vi "Fits_Create_Header.vi"(1 "Commentaire":string, 2 "Exptim":sgl, 3 "naxis3":i32=1, 4 "naxis2":i32, 5 "naxis1":i32, 6 "Type de données":T1) -> (0 "FITS header":string="SIMPLE  =                    T / Std FITS                                       BITPIX  =                    8 / NBER OF BITS PER PIXEL                         NAXIS   =                    2 / NBER OF AXIS                                   NAXIS1  =                    0 / FIRST VARYING AXIS                             NAXIS2  =                    0 / SECOND VARYING AXIS                            BZERO   =                    0 / DATA = BSCALE * DATA + BZERO                   BSCALE  =                    1 / DATA = BSCALE * DATA + BZERO                   DATE    =           11/03/2013 / LOCAL DATE dd/mm/yyyy                          TIME    =             11:26:53 / LOCAL TIME hh:mm:ss                            EXPTIM  =             0,000000 / INTEGRATION TIME  s                            NOM_PATI=               Durand / Nom du patient                                 COMMENT =                                                                                                                                                                                                                                       END                                                                                                                                                                                                                                                                                                                                                                                                                                                                                                                                                                                                                                                                                                                                                                                                                                                                                                                                                                                                                                                                                                                                                                                                                                                                                                                                                                                                                                                                                                                                                                                                                                                                                                                                                                                                                             ")   [LabVIEW 2020]
doc: "Creates the header string (multiple of 2880 characters) for a FITS image.\n\nThe dimensions of the data cube must be provided in input : they are naxis1, naxis2, naxis3. For a single image, set naxis3 to 1 (or any integer value less or equal to 1).\n\nThe data-types are:\n0 for U8 (unsigned 8bit)\n1 for I16 (signed integer 16bit)\n2 for I32 (signed integer 32bit)\n3 for SGL (float 32bit)\n4 for DBL(float 64bit)\n5 for complex (2xfloat 64bit)"
uses:
  DataTyp_Header.ctl
panel:
  in  "NomChamp":string="NOM_PATI"
  in  "Commentaire":string="Nom du patient"
  in  "VeleuChamp 1":string="Durand"
  out "FITS header 2":string
  in  "length (rest)":i32
  out "nb char header":i32=2880
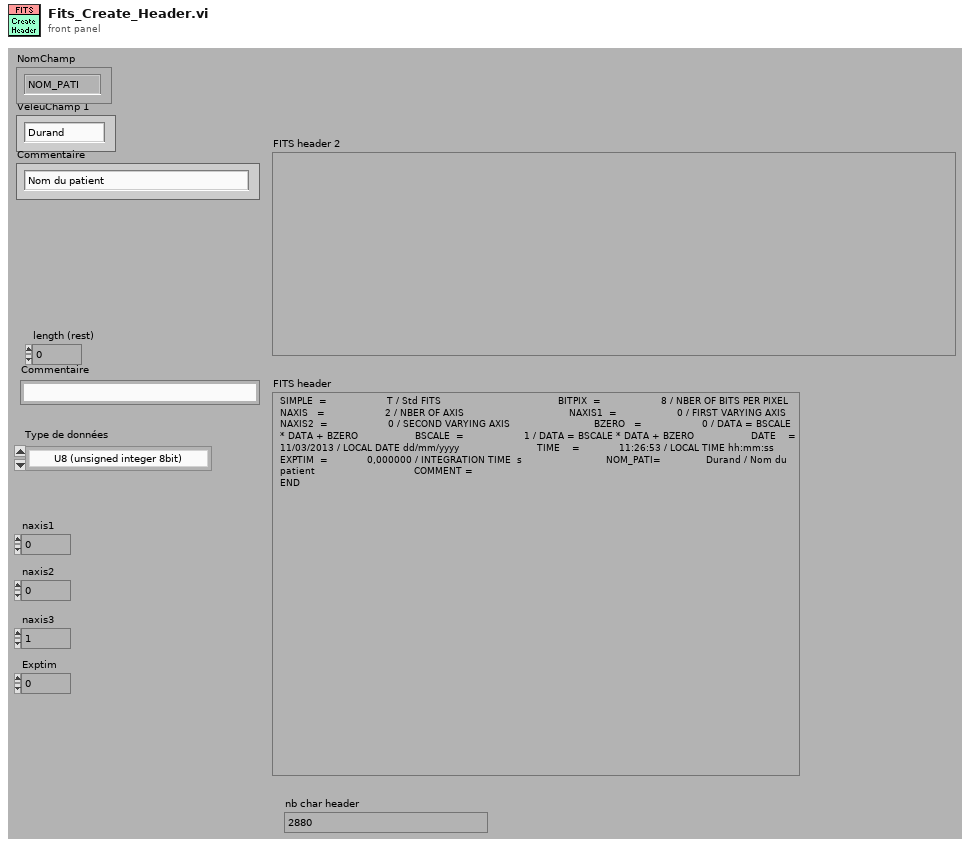
[diagram p1: front panel]
types:
  T1 = typedef "DataTyp_Header.ctl" = enum16{"U8 (unsigned integer 8bit)", "I16 (signed integer 16bit)", "U16 (unsigned integer 16 bit)", "I32 (signed integer 32bit)", "U32 (unsigned integer 32 bit)", "SGL (float 32bit)", "DBL(float 64bit)", "complex (2xfloat 64bit)"}
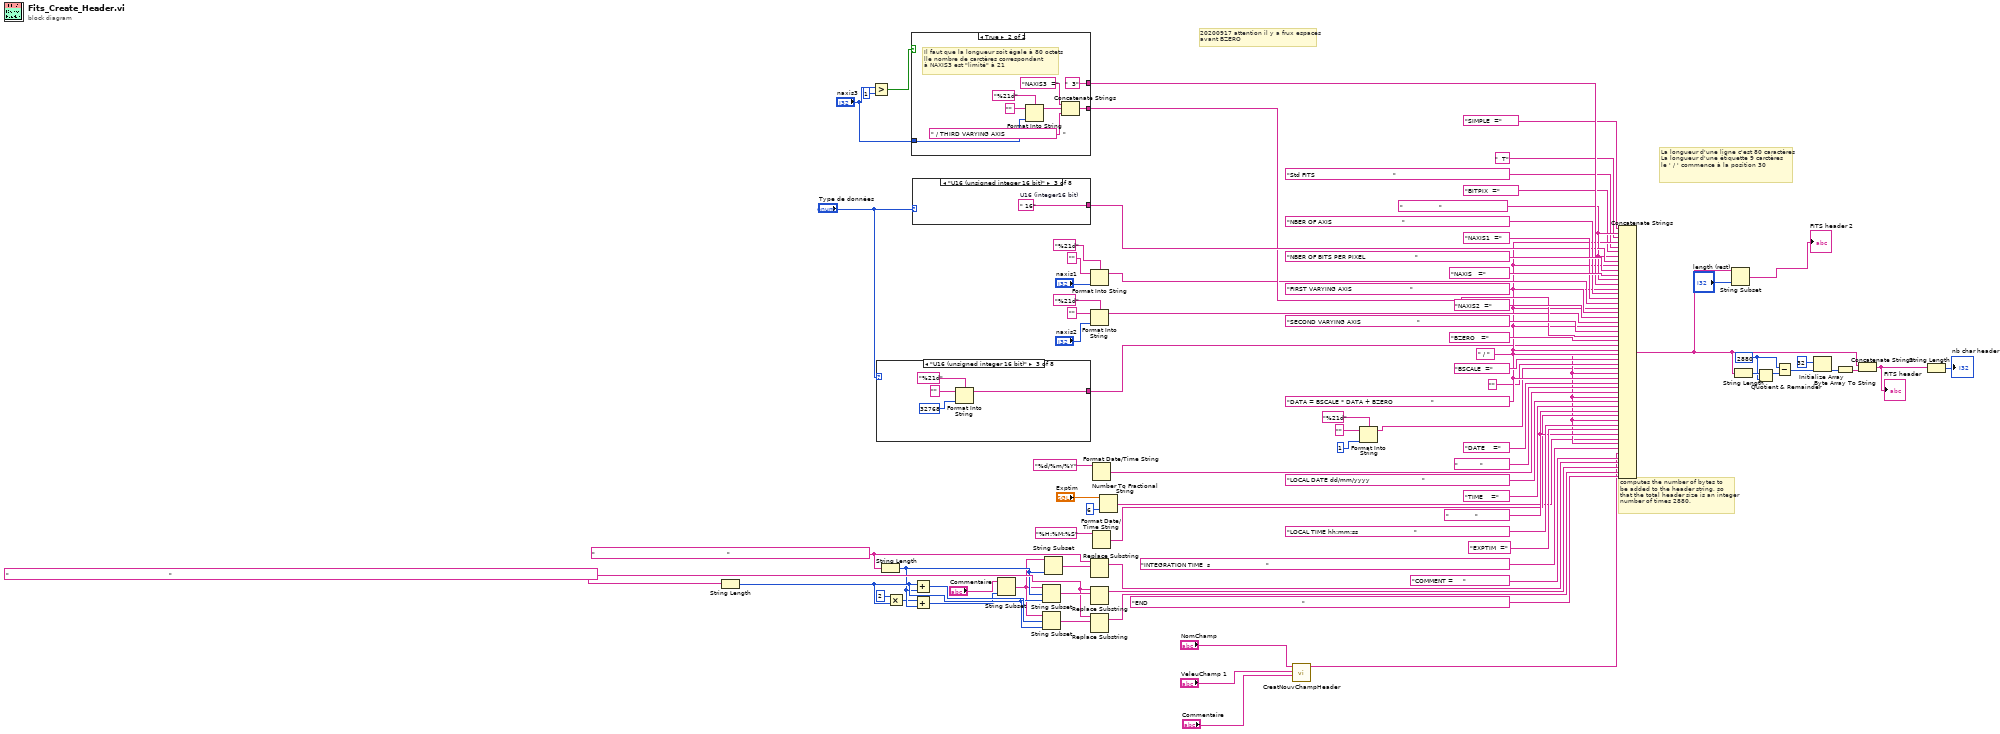
[diagram p0: block diagram]
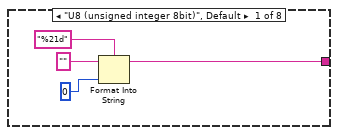
[diagram p2: hidden frame]
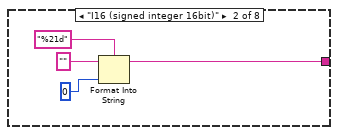
[diagram p3: hidden frame]
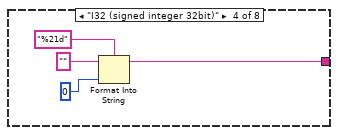
[diagram p4: hidden frame]
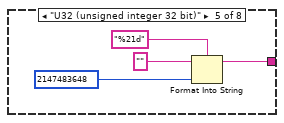
[diagram p5: hidden frame]
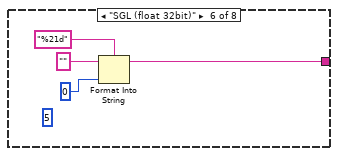
[diagram p6: hidden frame]
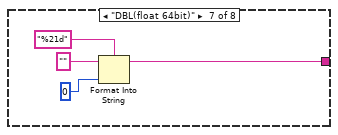
[diagram p7: hidden frame]
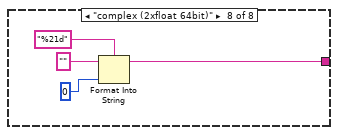
[diagram p8: hidden frame]
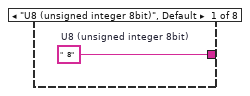
[diagram p9: hidden frame]
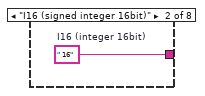
[diagram p10: hidden frame]
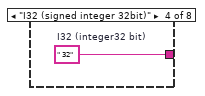
[diagram p11: hidden frame]
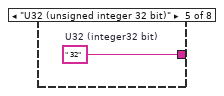
[diagram p12: hidden frame]
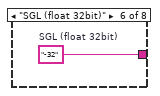
[diagram p13: hidden frame]
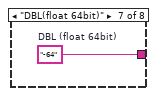
[diagram p14: hidden frame]
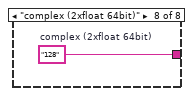
[diagram p15: hidden frame]
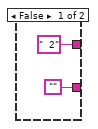
[diagram p16: hidden frame]
diagram:
  w51 = "                                                                                " ("chaîne")
  w55 = "                                                                  " ("chaîne")
  w26 = "             "
  w62 = "DATA = BSCALE * DATA + BZERO                   " ("Sous-chaîne")
  w76 = 2880 ("y")
  w16 = " / "
  w18 = "                  "
  # "20200917 attention il y a frux espaces \navant BZERO"
  # "La longueur d'une ligne c'est 80 caractères\nLa longueur d'une étiquette 9 carctères\nle ' / ' commence à la position 30"
  # "computes the number of bytes to\nbe added to the header string, so \nthat the total header size is an integer\nnumber of times 2880."
  n1 = String Length(string=w51) -> (length=w46:i32)
  n2 = Greater?(x="naxis3", y=1) -> (0:w78:bool)
  n3 = case shown="\"U16 (unsigned integer 16 bit)\"" "Type de données" {
    tunnel: [w87 w91 w95 w99 w103 w107 w111 w115] -> w5
    frame "U8 (unsigned integer 8bit)", Default {
      n4 = Format Into String(format string="%21d" ("chaîne de format"), initial string="" ("chaîne initiale"), u32 0 ("Nouvel élément")) -> (resulting string=w87:string)  [unwired: 1 in, 1 out]
    }
    frame "I16 (signed integer 16bit)" {
      n5 = Format Into String(format string="%21d" ("chaîne de format"), initial string="" ("chaîne initiale"), u32 0 ("Nouvel élément")) -> (resulting string=w91:string)  [unwired: 1 in, 1 out]
    }
    frame "U16 (unsigned integer 16 bit)" {
      n6 = Format Into String(format string="%21d" ("chaîne de format"), initial string="" ("chaîne initiale"), 32768 ("Nouvel élément")) -> (resulting string=w95:string)  [unwired: 1 in, 1 out]
    }
    frame "I32 (signed integer 32bit)" {
      n7 = Format Into String(format string="%21d" ("chaîne de format"), initial string="" ("chaîne initiale"), u32 0 ("Nouvel élément")) -> (resulting string=w99:string)  [unwired: 1 in, 1 out]
    }
    frame "U32 (unsigned integer 32 bit)" {
      n8 = Format Into String(format string="%21d" ("chaîne de format"), initial string="" ("chaîne initiale"), u32 2147483648 ("Nouvel élément")) -> (resulting string=w103:string)  [unwired: 1 in, 1 out]
    }
    frame "SGL (float 32bit)" {
      (unwired) i16 5 ("largeur (-)")
      n9 = Format Into String(format string="%21d" ("chaîne de format"), initial string="" ("chaîne initiale"), u32 0 ("Nouvel élément")) -> (resulting string=w107:string)  [unwired: 1 in, 1 out]
    }
    frame "DBL(float 64bit)" {
      n10 = Format Into String(format string="%21d" ("chaîne de format"), initial string="" ("chaîne initiale"), u32 0 ("Nouvel élément")) -> (resulting string=w111:string)  [unwired: 1 in, 1 out]
    }
    frame "complex (2xfloat 64bit)" {
      n11 = Format Into String(format string="%21d" ("chaîne de format"), initial string="" ("chaîne initiale"), u32 0 ("Nouvel élément")) -> (resulting string=w115:string)  [unwired: 1 in, 1 out]
    }
  }
  n12 = String Length(string=w55) -> (length=w45:i32)
  n13 = Multiply(x=i16 2 ("y"), y=w46) -> (x*y=w44:i32)
  n14 = case shown="True" w78 {
    tunnel: ["  2" "  3"] -> w83
    tunnel: ["" w125] -> w39
    tunnel: "naxis3" -> [_ w123]
    frame False {
    }
    frame True {
      # "Il faut que la longueur soit égale à 80 octets\nlle nombre de carctères correspondant\nà NAXIS3 est \"limité\" à 21"
      n15 = Format Into String(format string="%21d" ("chaîne de format"), initial string="" ("chaîne initiale"), w123) -> (resulting string=w122:string)  [unwired: 1 in, 1 out]
      n16 = Concatenate Strings("NAXIS3  =" ("Sous-chaîne"), w122, " / THIRD VARYING AXIS                             " ("Sous-chaîne")) -> (w125:string)
    }
  }
  n17 = case shown="\"U16 (unsigned integer 16 bit)\"" "Type de données" {
    tunnel: [w129 w130 w131 w132 w133 w134 w135 w136] -> w59
    frame "U8 (unsigned integer 8bit)", Default {
      w129 = "  8"  # U8 (unsigned integer 8bit)
    }
    frame "I16 (signed integer 16bit)" {
      w130 = " 16"  # I16 (integer 16bit)
    }
    frame "U16 (unsigned integer 16 bit)" {
      w131 = " 16"  # U16 (integer16 bit)
    }
    frame "I32 (signed integer 32bit)" {
      w132 = " 32"  # I32 (integer32 bit)
    }
    frame "U32 (unsigned integer 32 bit)" {
      w133 = " 32"  # U32 (integer32 bit)
    }
    frame "SGL (float 32bit)" {
      w134 = "-32"  # SGL (float 32bit)
    }
    frame "DBL(float 64bit)" {
      w135 = "-64"  # DBL (float 64bit)
    }
    frame "complex (2xfloat 64bit)" {
      w136 = "128"  # complex (2xfloat 64bit)
    }
  }
  n18 = Add(x=w46, y=w45) -> (x+y=w49:i32)
  n19 = Add(x=w44, y=w45) -> (x+y=w43:i32)
  n20 = String Subset(string="Commentaire", length (rest)=w43) -> (substring=w41:string)  [unwired: 1 out]
  n21 = String Subset(string=w41, offset (0)=w45, length (rest)=w46) -> (substring=w53:string)
  n22 = String Subset(string=w41, offset (0)=w49, length (rest)=w46) -> (substring=w50:string)
  n23 = String Subset(string=w41, length (rest)=w45) -> (substring=w54:string)  [unwired: 1 out]
  n24 = Format Into String(format string="%21d" ("chaîne de format"), initial string="" ("chaîne initiale"), "naxis1") -> (resulting string=w34:string)  [unwired: 1 in, 1 out]
  n25 = Format Into String(format string="%21d" ("chaîne de format"), initial string="" ("chaîne initiale"), "naxis2") -> (resulting string=w30:string)  [unwired: 1 in, 1 out]
  n26 = Replace Substring(4:w54, 5:w55) -> (1:w20:string)  [unwired: 3 out]
  n27 = Replace Substring(4:w53, 5:w51) -> (1:w52:string)  [unwired: 3 out]
  n28 = Replace Substring(4:w50, 5:w51) -> (1:w48:string)  [unwired: 3 out]
  n29 = Format Date/Time String(time format string (%c)="%d/%m/%Y" ("chaîne de format de l'heure (%c)")) -> (date/time string=w56:string)  [unwired: 2 out]
  n30 = Format Date/Time String(time format string (%c)="%H:%M:%S" ("chaîne de format de l'heure (%c)")) -> (date/time string=w25:string)  [unwired: 2 out]
  n31 = Number To Fractional String(number="Exptim", precision (6)=i16 6 ("width (-)")) -> (F-format string=w10:string)  [unwired: 2 in]
  n32 = call "CreatNouvChampHeader.vi"("CommentairChamp"="Commentaire", "ValChamp"="VeleuChamp 1", "NomChamp"="NomChamp") -> ("ChampHeader"=w9:string)  [unwired: 8 in]
  n33 = Format Into String(format string="%21d" ("chaîne de format"), initial string="" ("chaîne initiale"), 1 ("Nouvel élément")) -> (resulting string=w2:string)  [unwired: 1 in, 1 out]
  n34 = Concatenate Strings("SIMPLE  =", w18, "  T", w16, "Std FITS                                       ", "BITPIX  =", w18, w59, w16, "NBER OF BITS PER PIXEL                         " ("Sous-chaîne"), "NAXIS   =" ("Sous-chaîne"), w18, w83, w16, "NBER OF AXIS                                   " ("Sous-chaîne"), "NAXIS1  =" ("Sous-chaîne"), w34, w16, "FIRST VARYING AXIS                             " ("Sous-chaîne"), "NAXIS2  =" ("Sous-chaîne"), w30, w16, "SECOND VARYING AXIS                            " ("Sous-chaîne"), w39, "BZERO   =" ("Sous-chaîne"), w5, w16, w62, "BSCALE  =" ("Sous-chaîne"), "" ("Sous-chaîne"), w2, w16, w62, "DATE    =" ("Sous-chaîne"), "           ", w56, w16, "LOCAL DATE dd/mm/yyyy                          " ("Sous-chaîne"), "TIME    =" ("Sous-chaîne"), w26, w25, w16, "LOCAL TIME hh:mm:ss                            " ("Sous-chaîne"), "EXPTIM  =" ("Sous-chaîne"), w26, w10, w16, "INTEGRATION TIME  s                            " ("Sous-chaîne"), w9, "COMMENT =     ", w20, w52, w48, "END                                                                             " ("Sous-chaîne")) -> (w13:string)
  n35 = String Subset(string=w13, length (rest)="length (rest)") -> (substring=→"FITS header 2":string)  [unwired: 1 in]
  n36 = String Length(string=w13) -> (length=w77:i32)
  n37 = Quotient & Remainder(x=w77, y=w76) -> (x-y*floor(x/y)=w75:i32)  [unwired: 1 out]
  n38 = Subtract(x=w76, y=w75) -> (x-y=w73:i32)
  n39 = Initialize Array(u8 32 ("Nouvel élément"), w73) -> (w72:u8[])
  n40 = Byte Array To String(unsigned byte array=w72) -> (string=w71:string)
  n41 = Concatenate Strings(w13, w71) -> (w61:string)
  "FITS header" <- w61
  n42 = String Length(string=w61) -> (length=→"nb char header":i32)
